vi "Intake Teleop.vi"(10 "Right Trigger":dbl, 11 "Left Trigger":dbl) -> ()   [LabVIEW 2018]
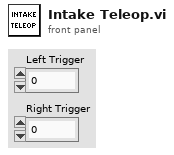
[diagram p1: front panel]
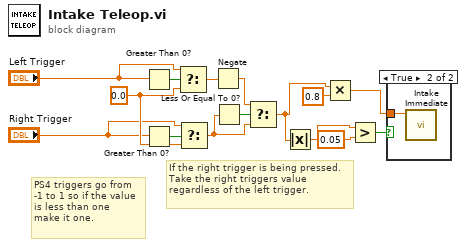
[diagram p0: block diagram]
diagram:
  w8 = 0.0
  # "PS4 triggers go from\n-1 to 1 so if the value\nis less than one\nmake it one."
  # "If the right trigger is being pressed. Take the right triggers value regardless of the left trigger."
  n1 = Greater Than 0?(x="Left Trigger") -> (x > 0?=w11:bool)
  n2 = Greater Than 0?(x="Right Trigger") -> (x > 0?=w9:bool)
  n3 = Select(t="Left Trigger", s=w11, f=w8) -> (s? t:f=w12:dbl)
  n4 = Select(t="Right Trigger", s=w9, f=w8) -> (s? t:f=w5:dbl)
  n5 = Negate(x=w12) -> (-x=w15:dbl)
  n6 = Less Or Equal To 0?(x=w5) -> (x <= 0?=w6:bool)
  n7 = Select(t=w15, s=w6, f=w5) -> (s? t:f=w2:dbl)
  n8 = Absolute Value(x=w2) -> (abs(x)=w1:dbl)
  n9 = Multiply(x=w2, y=0.8) -> (x*y=w3:dbl)
  n10 = Greater?(x=w1, y=0.05) -> (0:w14:bool)
  n11 = case shown="True" w14 {
    tunnel: w3 -> [_ w16]
    frame False {
    }
    frame True {
      n12 = call "Intake Immediate.vi"("Speed"=w16) -> ()  [unwired: 10 in, 1 out]
    }
  }
